vi "KE2260B Special Read.vi"(8 "error in (no error)":errorcluster, 10 "byte count":u32, 11 "VISA session":refnum<visa-resource-name>) -> (0 "error out":errorcluster, 1 "Return Count":u32, 2 "read buffer":string, 3 "dup VISA session":refnum<visa-resource-name>)   [LabVIEW 2021, in "Keithley 2260B.lvlib"]
uses:
  Keithley 2260B.lvlib
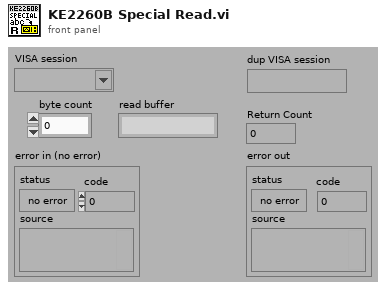
[diagram p1: front panel]
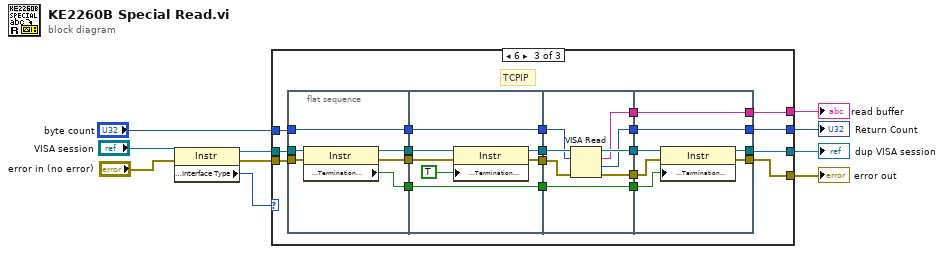
[diagram p0: block diagram]
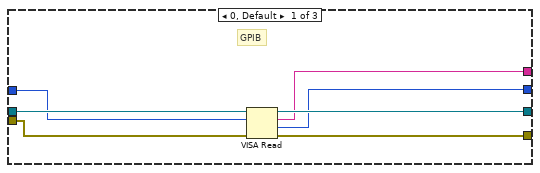
[diagram p2: hidden frame]
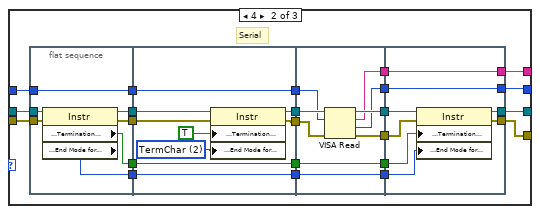
[diagram p3: hidden frame]
diagram:
  n1 = property class="Instr"(reference="VISA session", error in="error in (no error)") -> (reference out=w10:refnum<visa-resource-name>, error out=w9:errorcluster, "Interface Information:Interface Type"=w1:u16)
  n2 = case shown="6" w1 {
    tunnel: w10 -> [w17 w40 w75]
    tunnel: w9 -> [w15 w39 w74]
    tunnel: [w12 w25 w78] -> w3
    tunnel: [w16 w24 w77] -> w6
    tunnel: [w14 w23 w76] -> w5
    tunnel: [w11 w22 w79] -> w7
    tunnel: "byte count" -> [w13 w20 w80]
    frame 0, Default {
      # "GPIB"
      n3 = VISA Read(VISA resource name=w17, byte count=w13, error in (no error)=w15) -> (VISA resource name out=w16:refnum<visa-resource-name>, read buffer=w12:string, return count=w11:u32, error out=w14:errorcluster)
    }
    frame 4 {
      # "Serial"
      n4 = flat-sequence {
        tunnel: w40 -> [w47]
        tunnel: w39 -> [w46]
        tunnel: [w45] -> w38
        tunnel: [w44] -> w37
        tunnel: [w43] -> w30
        tunnel: [w42] -> w27
        tunnel: w20 -> [w41]
        tunnel: [w41] -> w18
        tunnel: w38 -> [w56]
        tunnel: w37 -> [w55]
        tunnel: [w52] -> w36
        tunnel: [w51] -> w35
        tunnel: [w50] -> w31
        tunnel: w30 -> [w50]
        tunnel: [w49] -> w28
        tunnel: w27 -> [w49]
        tunnel: [w48] -> w19
        tunnel: w18 -> [w48]
        tunnel: w36 -> [w65]
        tunnel: w35 -> [w64]
        tunnel: [w63] -> w34
        tunnel: [w62] -> w33
        tunnel: [w61] -> w32
        tunnel: w31 -> [w61]
        tunnel: [w60] -> w29
        tunnel: w28 -> [w60]
        tunnel: [w59] -> w26
        tunnel: [w58] -> w21
        tunnel: w19 -> [w57]
        tunnel: w34 -> [w73]
        tunnel: w33 -> [w72]
        tunnel: w32 -> [w71]
        tunnel: w29 -> [w70]
        tunnel: [w69] -> w25
        tunnel: w26 -> [w69]
        tunnel: [w68] -> w24
        tunnel: [w67] -> w23
        tunnel: [w66] -> w22
        tunnel: w21 -> [w66]
        frame #0 {
          n5 = property class="Instr"(reference=w47, error in=w46) -> (reference out=w45:refnum<visa-resource-name>, error out=w44:errorcluster, "Message Based Settings:Termination Character Enable"=w43:bool, "Serial Settings:End Mode for Reads"=w42:u16)
        }
        frame #1 {
          w53 = u16 2 items=["None", "LastBit", "TermChar"] ("Serial Settings:Serial End Mode for Reads")
          n6 = property class="Instr"(reference=w56, error in=w55, "Message Based Settings:Termination Character Enable"=TRUE, "Serial Settings:End Mode for Reads"=w53) -> (reference out=w52:refnum<visa-resource-name>, error out=w51:errorcluster)
        }
        frame #2 {
          n7 = VISA Read(VISA resource name=w65, byte count=w57, error in (no error)=w64) -> (VISA resource name out=w63:refnum<visa-resource-name>, read buffer=w59:string, return count=w58:u32, error out=w62:errorcluster)
        }
        frame #3 {
          n8 = property class="Instr"(reference=w73, error in=w72, "Message Based Settings:Termination Character Enable"=w71, "Serial Settings:End Mode for Reads"=w70) -> (reference out=w68:refnum<visa-resource-name>, error out=w67:errorcluster)
        }
      }
    }
    frame 6 {
      # "TCPIP"
      n9 = flat-sequence {
        tunnel: w75 -> [w99]
        tunnel: w74 -> [w98]
        tunnel: [w97] -> w93
        tunnel: [w96] -> w92
        tunnel: [w95] -> w91
        tunnel: w80 -> [w94]
        tunnel: [w94] -> w90
        tunnel: w93 -> [w106]
        tunnel: w92 -> [w105]
        tunnel: [w103] -> w89
        tunnel: [w102] -> w88
        tunnel: [w101] -> w87
        tunnel: w91 -> [w101]
        tunnel: [w100] -> w86
        tunnel: w90 -> [w100]
        tunnel: w89 -> [w114]
        tunnel: w88 -> [w113]
        tunnel: [w112] -> w85
        tunnel: [w111] -> w84
        tunnel: [w110] -> w83
        tunnel: w87 -> [w110]
        tunnel: [w109] -> w82
        tunnel: [w108] -> w81
        tunnel: w86 -> [w107]
        tunnel: w85 -> [w121]
        tunnel: w84 -> [w120]
        tunnel: w83 -> [w119]
        tunnel: [w118] -> w78
        tunnel: w82 -> [w118]
        tunnel: [w117] -> w77
        tunnel: [w116] -> w76
        tunnel: [w115] -> w79
        tunnel: w81 -> [w115]
        frame #0 {
          n10 = property class="Instr"(reference=w99, error in=w98) -> (reference out=w97:refnum<visa-resource-name>, error out=w96:errorcluster, "Message Based Settings:Termination Character Enable"=w95:bool)
        }
        frame #1 {
          n11 = property class="Instr"(reference=w106, error in=w105, "Message Based Settings:Termination Character Enable"=TRUE) -> (reference out=w103:refnum<visa-resource-name>, error out=w102:errorcluster)
        }
        frame #2 {
          n12 = VISA Read(VISA resource name=w114, byte count=w107, error in (no error)=w113) -> (VISA resource name out=w112:refnum<visa-resource-name>, read buffer=w109:string, return count=w108:u32, error out=w111:errorcluster)
        }
        frame #3 {
          n13 = property class="Instr"(reference=w121, error in=w120, "Message Based Settings:Termination Character Enable"=w119) -> (reference out=w117:refnum<visa-resource-name>, error out=w116:errorcluster)
        }
      }
    }
  }
  "dup VISA session" <- w6
  "error out" <- w5
  "Return Count" <- w7
  "read buffer" <- w3
